vi "Modbus Items - Check Items Types Support.vi"(8 "error in (no error)":errorcluster, 10 "Modbus_Type":i32(ring) items=["Master", "Slave"], 11 "Modbus Items In":T1[](array[typedef])) -> (0 "error out":errorcluster, 3 "Modbus Items Out":T1[](array[typedef]))   [LabVIEW 2014, in "Modbus System Explorer.lvlib"]
uses:
  Modbus System Explorer.lvlib
  XML Deserializer/XML VIs/API/Controls/Modbus_Items.ctl
  XML Deserializer/XML VIs/API/Controls/Modbus_Item_Type.ctl
  Shared/Modbus Shared.lvlib
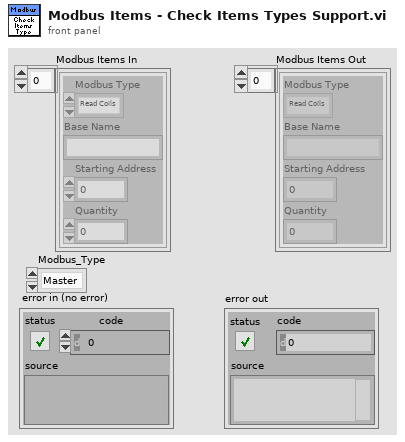
[diagram p1: front panel]
types:
  T1 = typedef "Modbus Shared.lvlib/Modbus_Items.ctl" = cluster{"Modbus Type":T2, "Base Name":string, "Starting Address":u16, "Quantity":u16}
  T2 = typedef "Modbus Shared.lvlib/Modbus_Item_Type.ctl" = enum16{"Read Coils", "Read Discrete Inputs", "Read Holding Registers", "Read Input Registers", "Write Multiple Coils", "Write Multiple Holding Registers", "Write Single Coil", "Write Single Holding Register", "Write Multiple Discrete Inputs", "Write Multiple Input Registers"}
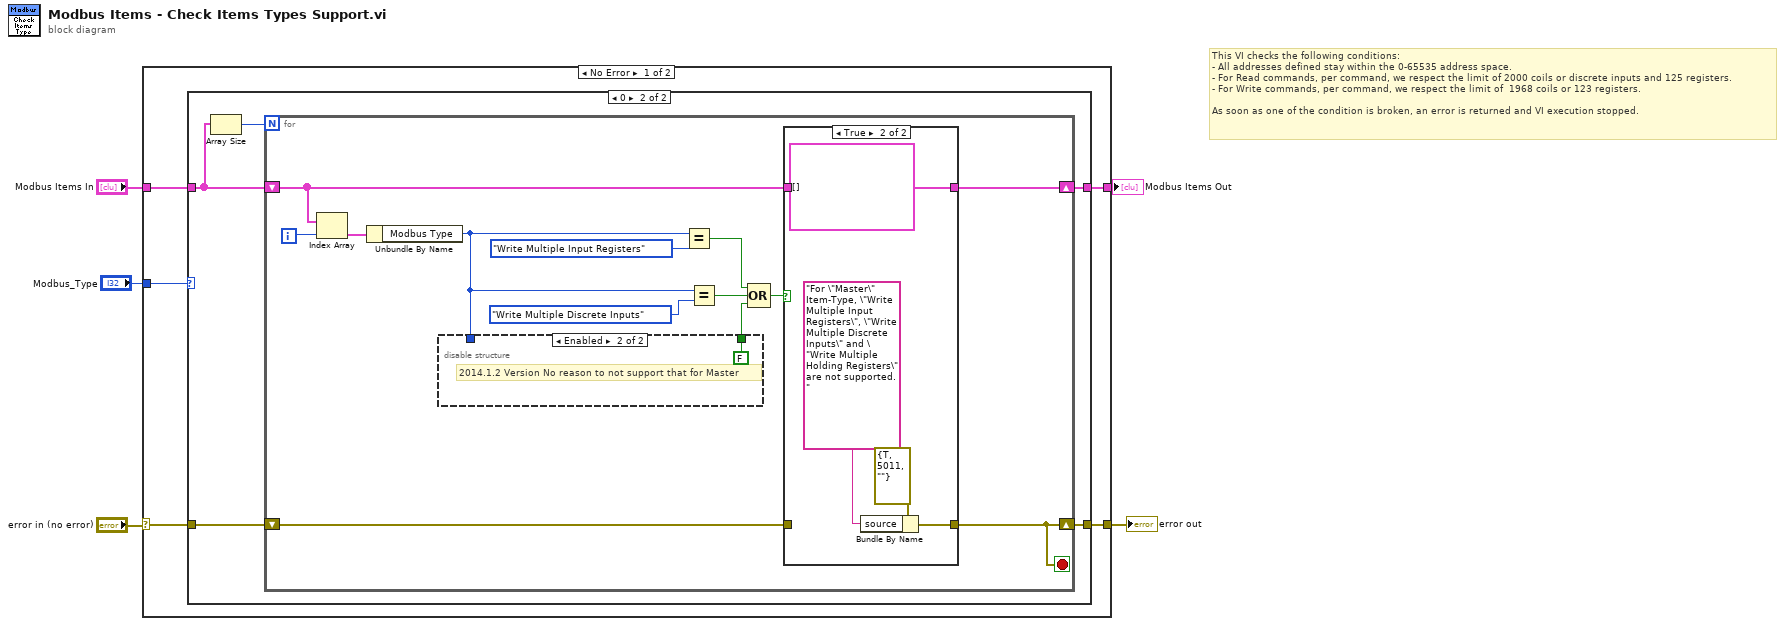
[diagram p0: block diagram]
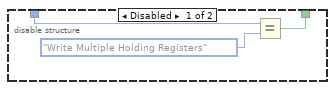
[diagram p3: hidden frame]
diagram:
  # "This VI checks the following conditions:\n- All addresses defined stay within the 0-65535 address space.\n- For Read commands, per command, we respect the limit of 2000 coils or discrete inputs and 125 registers.\n- For Write commands, per command, we respect the limit of  1968 coils or 123 registers.\n\nAs soon as one of the condition is broken, an error is returned and VI execution stopped."
  n1 = case shown="No Error" "error in (no error)" {
    selector: "error in (no error)" -> [w10 w42]
    tunnel: [w9 w42] -> w4
    tunnel: "Modbus Items In" -> [w7 w41]
    tunnel: [w8 w41] -> w2
    tunnel: "Modbus_Type" -> [w6 _]
    frame No Error {
      n2 = case shown="0" w6 {
        tunnel: w10 -> [w11 w17]
        tunnel: [w11 w16] -> w9
        tunnel: [w12 w15] -> w8
        tunnel: w7 -> [w12 w13]
        frame 1, Default {
        }
        frame 0 {
          n3 = Array Size(array=w13) -> (size(s)=w14:i32)
          n4 = for {
            N: w14 -> [_]
            shift-right: [w28] -> w16
            shift-left: w17 -> [w30]
            shift-right: [w29] -> w15
            shift-left: w13 -> [w26]
            i -> [w25]
            stop <- w28 stop-if-true
            n5 = Index Array(array=w26, index=w25) -> (element=w24:T1)
            n6 = Unbundle By Name(w24) -> ("Modbus Type"=w21:T2)
            n7 = disable-structure shown="Enabled" {
              disable-tunnel: w21 -> [w32 _]
              disable-tunnel: [w31 FALSE] -> w18
              frame Disabled {
                n8 = Equal?(x=w32, y=Modbus_Item_Type."Write Multiple Holding Registers") -> (x = y?=w31:bool)
              }
              frame Enabled {
                # "2014.1.2 Version No reason to not support that for Master"
              }
            }
            n9 = Equal?(x=w21, y=Modbus_Item_Type."Write Multiple Input Registers") -> (x = y?=w20:bool)
            n10 = Equal?(x=w21, y=Modbus_Item_Type."Write Multiple Discrete Inputs") -> (x = y?=w19:bool)
            n11 = Compound Arithmetic op=OR(w20, w19, w18) -> (w27:bool)
            n12 = case shown="True" w27 {
              tunnel: w30 -> [w35 _]
              tunnel: w26 -> [w36 _]
              tunnel: [w36 T1[] [] ("Modbus Items In")] -> w29
              tunnel: [w35 w39] -> w28
              frame False {
              }
              frame True {
                n13 = Bundle By Name(cluster=errorcluster {"status"=TRUE, "code"=5011, "source"=""} ("error IO"), "source"="For \"Master\" Item-Type, \"Write Multiple Input Registers\", \"Write Multiple Discrete Inputs\" and \"Write Multiple Holding Registers\" are not supported.") -> (w39:errorcluster)
              }
            }
          }
        }
      }
    }
    frame Error {
    }
  }
  "error out" <- w4
  "Modbus Items Out" <- w2
